vi "Drive Controller.vi"(8 "error in":errorcluster) -> ()   [LabVIEW 2017]
doc: "This VI executes continuously carrying out the current operation and responding to updates or new operation requests. It will often contain the timing or control code that is difficult to place directly in TeleOp. This VI generally opens all sensors and motors and isolates the rest of the robot code from knowing implementation details of how the operations are carried out."
uses:
  <vilib>/Rock Robotics/WPI/Framework/Completion Status.ctl
  Drive Setpoints.ctl
  Drive Operations.ctl
  Shared/RobotNeededPathData.ctl
  <vilib>/Rock Robotics/WPI/SafetyOutput/WPI_SafetyOutputConfigMenu.ctl
  <vilib>/Rock Robotics/SystemInterfaces/DIO/FPGA_DIOPWMChannel.ctl
  <vilib>/Rock Robotics/SystemInterfaces/DIO/FPGA_DIOChannel.ctl
  <vilib>/Rock Robotics/WPI/DriverStation/WPI_DriverStationRobotMode2.ctl
  <vilib>/Rock Robotics/WPI/ThirdParty/Sensors/navX/_TypeDefs/FRIC_navX_DeviceNumbersTypeDef.ctl
  <extravilib>/ChannelInstances/Lossy Stream-c(dbl,dbl,dbl,c(dbl,dbl))/Write With Abort.vi
  <extravilib>/ChannelInstances/Lossy Stream-c(dbl,dbl,dbl,c(dbl,dbl))/Read With Abort.vi
  <extravilib>/ChannelInstances/Lossy Stream-c(dbl,dbl,dbl,c(dbl,dbl))/Endpoint.vi
  <extravilib>/ChannelInstances/Lossy Stream-c(dbl,dbl,dbl,c(dbl,dbl))/EndpointRead.vi
  <vilib>/Rock Robotics/WPI/RobotDrive/WPI_RobotDriveOpen4MotorWithSPARK.vi
  <vilib>/Rock Robotics/WPI/Counter/WPI_CounterDigitalInputToDigitalSource.vi
  <vilib>/Rock Robotics/WPI/RobotDrive/WPI_RobotDriveOpen2MotorWithSPARK.vi
  <extravilib>/ChannelInstances/Lossy Stream-c(dbl,dbl,dbl,c(dbl,dbl))/Instantiate.vi
  <extravilib>/ChannelInstances/Lossy Stream-c(dbl,dbl,dbl,c(dbl,dbl))/)Channel.vi
  <resource>/ChannelSupport/_ChannelSupport/WaitIfNeeded.vi
  <vilib>/addons/control/pid/pid.llb/PID (DBL).vi
  Configuration/Constants.vi
  <vilib>/Rock Robotics/Network Tables/NT Read Number.vi
  Framework/Robot Global Data.vi
  Drive Published Globals.vi
  <vilib>/addons/control/pid/NI_PID_pid.lvlib
  <extravilib>/ChannelInstances/Lossy Stream-c(dbl,dbl,dbl,c(dbl,dbl)).lvlib
panel:
  out "Waveform Chart":cluster{dbl, dbl}(graph)={180.0, 177.43}
  in  "Points":cluster{"X":dbl, "Y":dbl}[](array[cluster])=[{"X"=0.0, "Y"=0.0}, {"X"=0.01, "Y"=0.0}, {"X"=0.011, "Y"=0.3}, {"X"=1.0, "Y"=1.0}]
  in  "PID gains":T1={"proportional gain (Kc)"=0.003, "integral time (Ti, min)"=0.0, "derivative time (Td, min)"=0.0} {"derivative time (Td, min)" format="%#_9g"}
  out "Numeric":dbl
  out "Yaw 2":dbl=2.309999999999988
  in  "Gains":T2={"FFV"=0.0059, "FFA"=0.0019, "Vel PID"={"P"=0.01, "I"=0.0, "D"=0.0}}
  in  "Interactive Values":T3={"Operation"=enum."Turn to Angle", "Left Speed"=-0.27, "Right Speed"=0.27, "Duration"=2.0, "Speed"=0.0, "Start Angle"=0.0, "Target Angle"=180.0, "Distance (inch)"=0.0, "Start Point (inch)"=0.0, "RobotNeededPathData"={"Path"=[], "MaxVel"=0.0, "MaxAccel"=-1.0, "Backwards?"=FALSE, "PointSpacing"=0.0, "LookaheadDist"=0.0, "Speed/Curve"=1.8, "SlowDistanceAtEnd"=12.0, "SlowSpeed"=15.0}} {"RobotNeededPathData"."SlowSpeed" format="%#_13g"; "RobotNeededPathData"."SlowDistanceAtEnd" format="%#_13g"; "RobotNeededPathData"."Speed/Curve" format="%#_13g"}
  in  "Buttons":cluster{"Execute Cmd":bool, "Abort Cmd":bool}
  out "Command Timing":cluster{"Start Time (ms)":u32, "Iterations":i32}={"Start Time (ms)"=1728587, "Iterations"=0}
  out "Status":T6
  out "Setpoints":T7(graph)
  out "Current\nCmd":string="Started at  15:35:35.928\nDefault: Reserve,  L 0.0, R 0.0, D 0.000000"
  # "Tip: The graph shows the motor setpoints. It may also be helpful to observe inputs and sensor values.\nYou may also want to display tuning or debugging controls."
  # ".0088"
  # ".0017"
  # ".02"
  # "Interactive Command: You may fill in the settings for a command\nand schedule it with the Execute button. You can observe and abort\nany command while fine tuning the code for the controller."
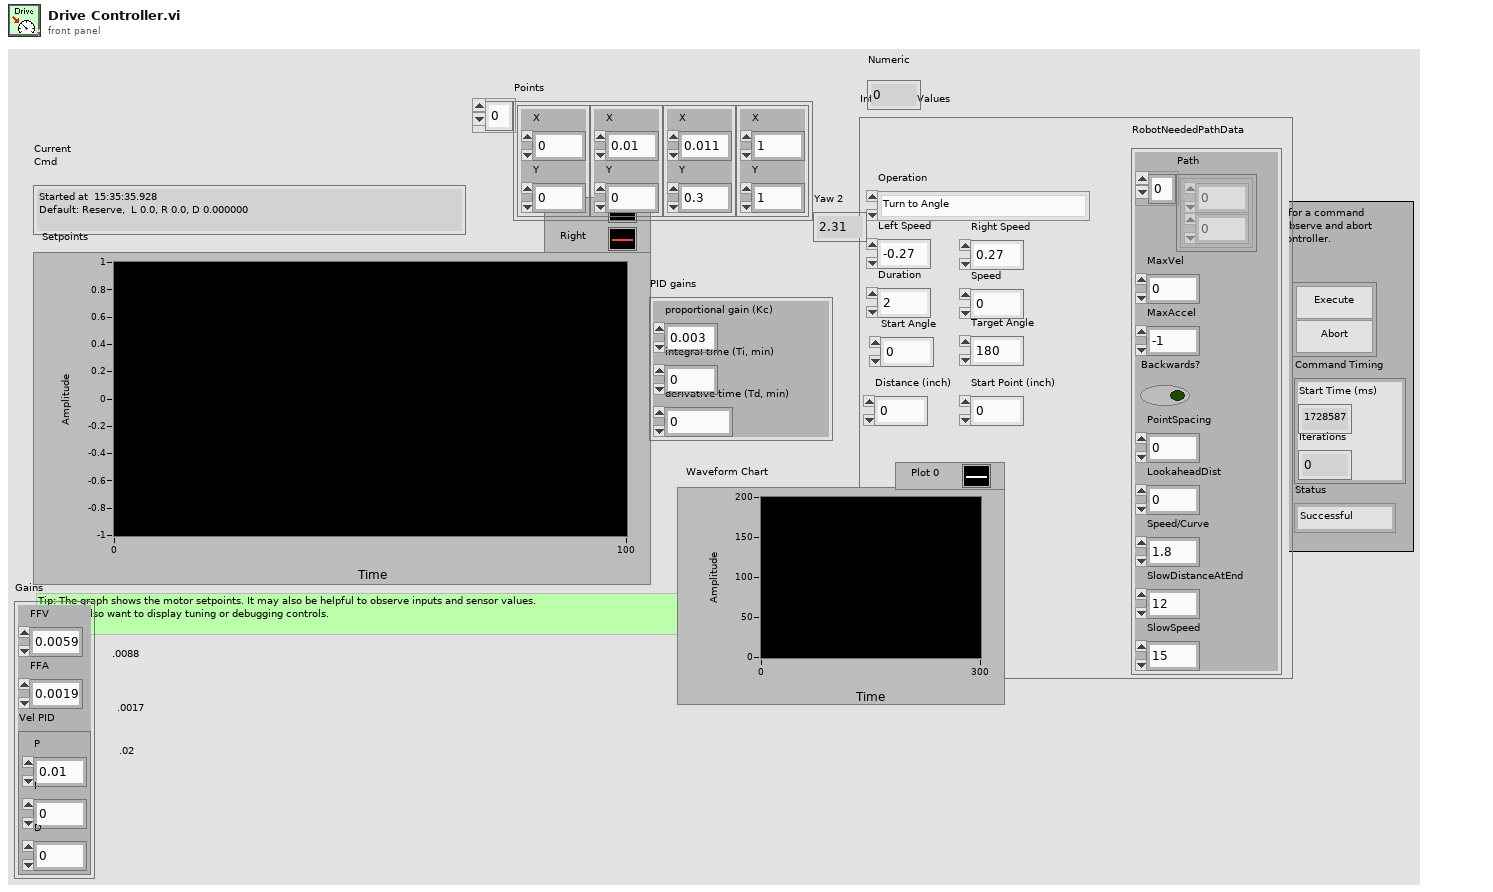
[diagram p1: front panel]
types:
  T1 = cluster{"proportional gain (Kc)":dbl, "integral time (Ti, min)":dbl, "derivative time (Td, min)":dbl}
  T2 = cluster{"FFV":dbl, "FFA":dbl, "Vel PID":cluster{"P":dbl, "I":dbl, "D":dbl}}
  T3 = typedef "Drive Setpoints.ctl" = cluster{"Operation":T4, "Left Speed":dbl, "Right Speed":dbl, "Duration":dbl, "Speed":dbl, "Start Angle":dbl, "Target Angle":dbl, "Distance (inch)":dbl, "Start Point (inch)":dbl, "RobotNeededPathData":T5}
  T4 = typedef "Drive Operations.ctl" = enum16{"Reserve", "Read Current", "Immediate", "Drive for Time", "Drive for Distance", "Turn to Angle", "Arc Turn", "Drive Path"}
  T5 = typedef "RobotNeededPathData.ctl" = cluster{"Path":cluster{dbl, dbl}[], "MaxVel":dbl, "MaxAccel":dbl, "Backwards?":bool, "PointSpacing":dbl, "LookaheadDist":dbl, "Speed/Curve":dbl, "SlowDistanceAtEnd":dbl, "SlowSpeed":dbl}
  T6 = typedef "Completion Status.ctl" = enum16{"Successful", "Aborted", "Incomplete"}
  T7 = cluster{"Left Setpoint":dbl, "Right Setpoint":dbl}
  T8 = typedef "FPGA_DIOChannel.ctl" = enum8{"DIO 0", "DIO 1", "DIO 2", "DIO 3", "DIO 4", "DIO 5", "DIO 6", "DIO 7", "DIO 8", "DIO 9", "DIO MXP 0", "DIO MXP 1", "DIO MXP 2", "DIO MXP 3", "DIO MXP 4", "DIO MXP 5", "DIO MXP 6", "DIO MXP 7", "DIO MXP 8", "DIO MXP 9", "DIO MXP 10", "DIO MXP 11", "DIO MXP 12", "DIO MXP 13", "DIO MXP 14", "DIO MXP 15", "SPI Port CS1", "SPI Port CS2", "SPI Port CS3", "SPI Port MISO", "SPI Port MOSI", "Invalid"}
  T9 = typedef "FPGA_DIOPWMChannel.ctl" = enum8{"PWM 0", "PWM 1", "PWM 2", "PWM 3", "PWM 4", "PWM 5", "PWM 6", "PWM 7", "PWM 8", "PWM 9", "PWM MXP 0", "PWM MXP 1", "PWM MXP 2", "PWM MXP 3", "PWM MXP 4", "PWM MXP 5", "PWM MXP 6", "PWM MXP 7", "PWM MXP 8", "PWM MXP 9", "Invalid"}
  T10 = typedef "WPI_SafetyOutputConfigMenu.ctl" = enum16{"Enable", "Disable"}
  T11 = typedef "WPI_DigitalInputDevRef.ctl" = cluster{"DevStatus":errorcluster, "DIO Channel":T8}
  T12 = typedef "FPGA_CounterEncoderSourceConvertionLVSourceType.ctl" = cluster{"DevStatus":errorcluster, "AnalogTriggerMode?":bool, "DigitalMode":cluster{"DIO Channel":T13}, "AnalogTriggerMode":cluster{"AnalogTriggerIndex":T14, "OutputType":T15}}
  T13 = typedef "FPGA_DIODigitalSourceChannel.ctl" = enum8{"DIO 0", "DIO 1", "DIO 2", "DIO 3", "DIO 4", "DIO 5", "DIO 6", "DIO 7", "DIO 8", "DIO 9", "DIO MXP 0", "DIO MXP 1", "DIO MXP 2", "DIO MXP 3", "DIO MXP 4", "DIO MXP 5", "DIO MXP 6", "DIO MXP 7", "DIO MXP 8", "DIO MXP 9", "DIO MXP 10", "DIO MXP 11", "DIO MXP 12", "DIO MXP 13", "DIO MXP 14", "DIO MXP 15", "Disabled"}
  T14 = typedef "FPGA_AnalogTriggerIndex.ctl" = enum8{"Trig 0", "Trig 1", "Trig 2", "Trig 3", "Trig 4", "Trig 5", "Trig 6", "Trig 7", "Invalid"}
  T15 = typedef "FPGA_AnalogTriggerOutType.ctl" = enum16{"InWindow", "TriggerState", "Rising", "Falling"}
  T16 = typedef "WPI_EncoderDevRef.ctl" = cluster{"DevStatus":errorcluster, "EncoderIndex":T17, "CounterIndex":T18, "DistancePerCount":dbl, "Decoding Type":T19}
  T17 = typedef "FPGA_EncoderIdx.ctl" = enum8{"Enc 0", "Enc 1", "Enc 2", "Enc 3", "Enc 4", "Enc 5", "Enc 6", "Enc 7", "Invalid"}
  T18 = typedef "FPGA_CounterCtrSystemIndex.ctl" = enum8{"Ctr 0", "Ctr 1", "Ctr 2", "Ctr 3", "Ctr 4", "Ctr 5", "Ctr 6", "Ctr 7", "Invalid"}
  T19 = typedef "WPI_EncoderType.ctl" = enum16{"1x", "2x", "4x"}
  T20 = typedef "WPI_RobotDriveDevRef.ctl" = cluster{"DevStatus":errorcluster, "Motors[]":T21[], "Square Inputs":bool, "Max Output":dbl}
  T21 = typedef "WPI_MotorControlDeviceRef.ctl" = cluster{"DeviceStatus":errorcluster, "Type":T22, "PWM":cluster{"PWM Channel":T9, "DeadBand":T23}, "CAN":cluster{"Device Number":u8, "SetOutput VI Ref":variant, "GetOutput VI Ref":variant, "Enable VI Ref":variant, "Disable VI Ref":variant, "Data":variant}, "Invert":bool, "DIO PWM":cluster{"PWM \"Enable\" Channel":T9, "DIOChannel":T8, "PWM Rate":dbl}}
  T22 = typedef "WPI_MotorControlType.ctl" = enum16{"PWM", "CAN", "DIO PWM"}
  T23 = typedef "WPI_PWMDeadband.ctl" = cluster{"Name":string, "maxPositivePwm":i32, "minPositivePwm":i32, "centerPwm":i32, "maxNegativePwm":i32, "minNegativePwm":i32, "angularRange":u16}
  T24 = typedef "Command Status Info.ctl" = cluster{"Name":string, "Status":T6, "notifier out":T25}
  T25 = typedef "Completion Notifier.ctl" = refnum<notifier>
  T26 = cluster{"SubSystem Data":T3, cluster{"Start Time (ms)":u32, "Iterations":i32}, cluster{"Command Info":T24, "Description":string, "Default Command":T3, "queue out":refnum<queue>, "Subsystem Name":string}}
  T27 = typedef "WPI_DriverStationRobotMode2.ctl" = enum16{"Autonomous Disabled", "Autonomous Enabled", "Teleop Disabled", "Teleop Enabled", "Disconnected", "Finish", "Test Disabled", "Test Enabled", "Emergency Stopped"}
  T28 = cluster{"Yaw":dbl, "Roll":dbl, "Pitch":dbl, "Heading":dbl, "Fused Heading":dbl}
  T29 = cluster{"dx/dt":dbl, "dx/dt":dbl, dbl, cluster{dbl, dbl}}
  T30 = typedef "Lossy Stream-c(dbl,dbl,dbl,c(dbl,dbl)).lvlib/)Channel.ctl" = refnum<queue>
  T31 = typedef "FRIC_navX_DeviceNumbersTypeDef.ctl" = enum16{"Dev0", "Dev1", "Dev2", "Dev3"}
  T32 = cluster{"LeftDistance":dbl, "RightDistance":dbl, "LeftVelocity":dbl, "RightVelocity":dbl, "Angle":dbl, "Location":cluster{dbl, dbl}}
  T33 = cluster{"dx/dt":dbl, "dx/dt":dbl, "Yaw":dbl, cluster{dbl, dbl}}
  T34 = cluster{"SubSystem Data":T3, cluster{"Start Time (ms)":u32, "Iterations":i32}, "Default Command Arguments":cluster{"Command Info":T24, "Description":string, "Default Command":T3, "queue out":refnum<queue>, "Subsystem Name":string}}
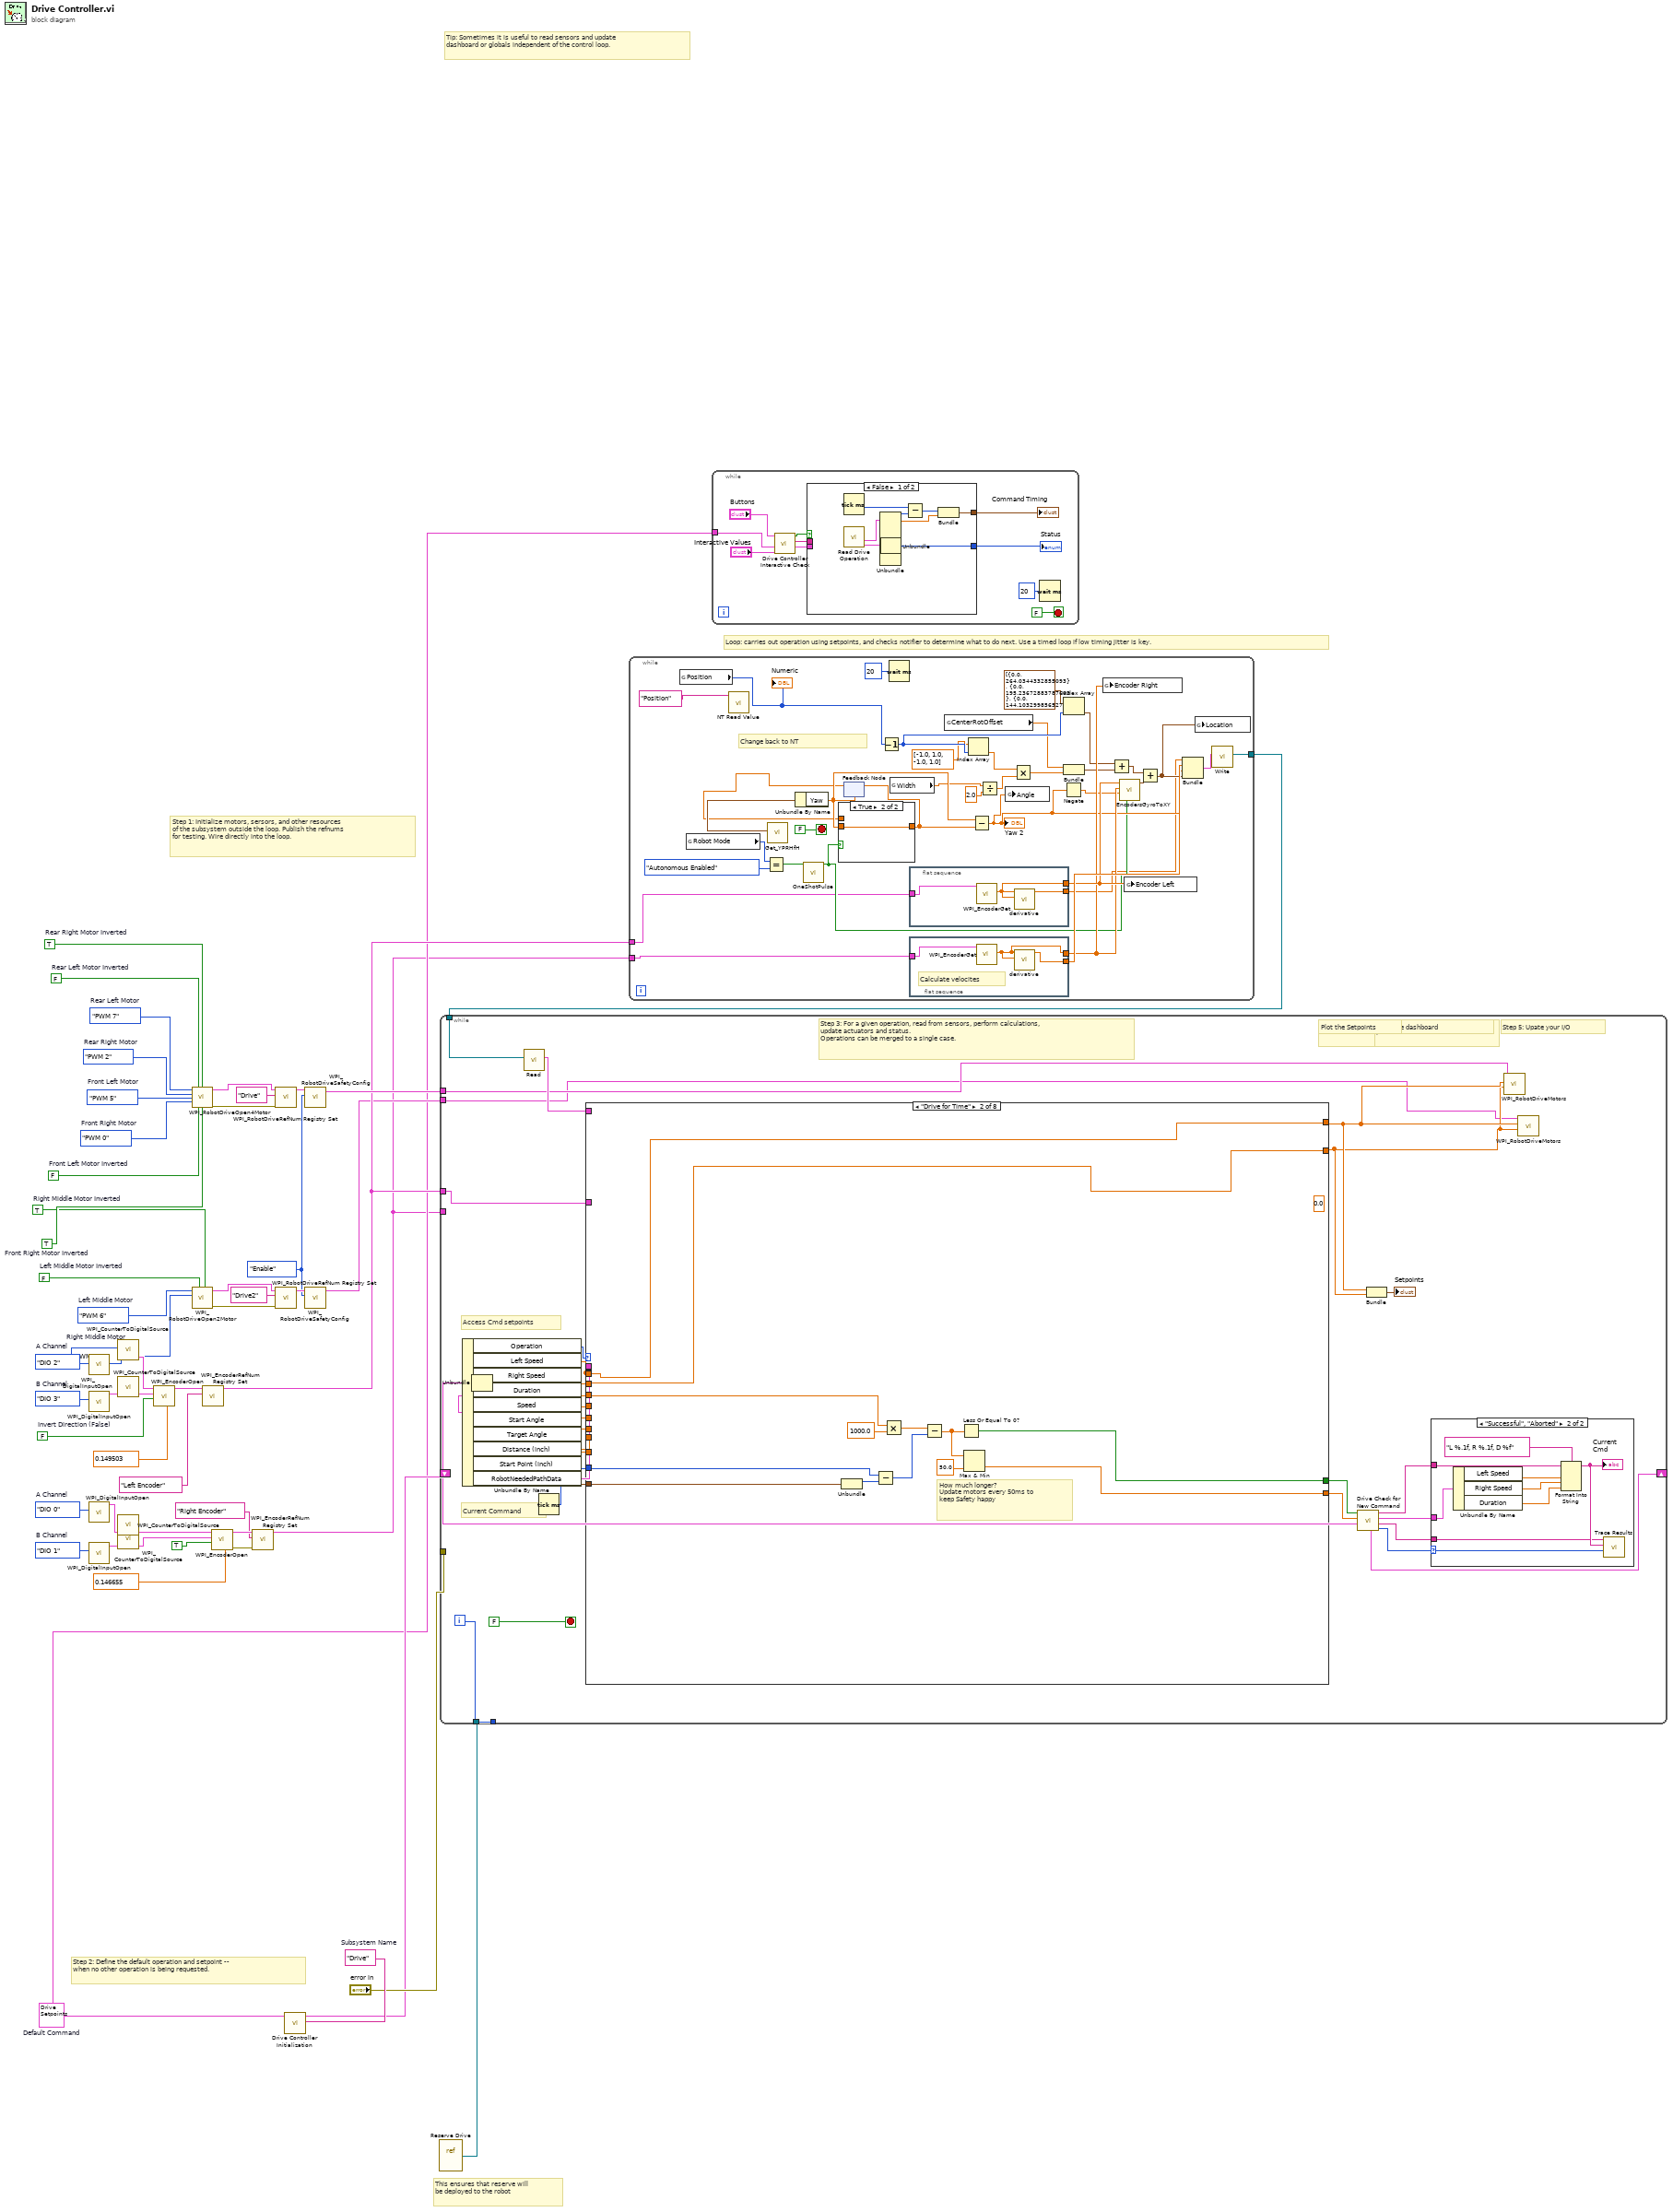
[diagram p0: block diagram]
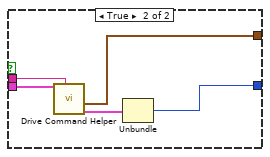
[diagram p3: hidden frame]
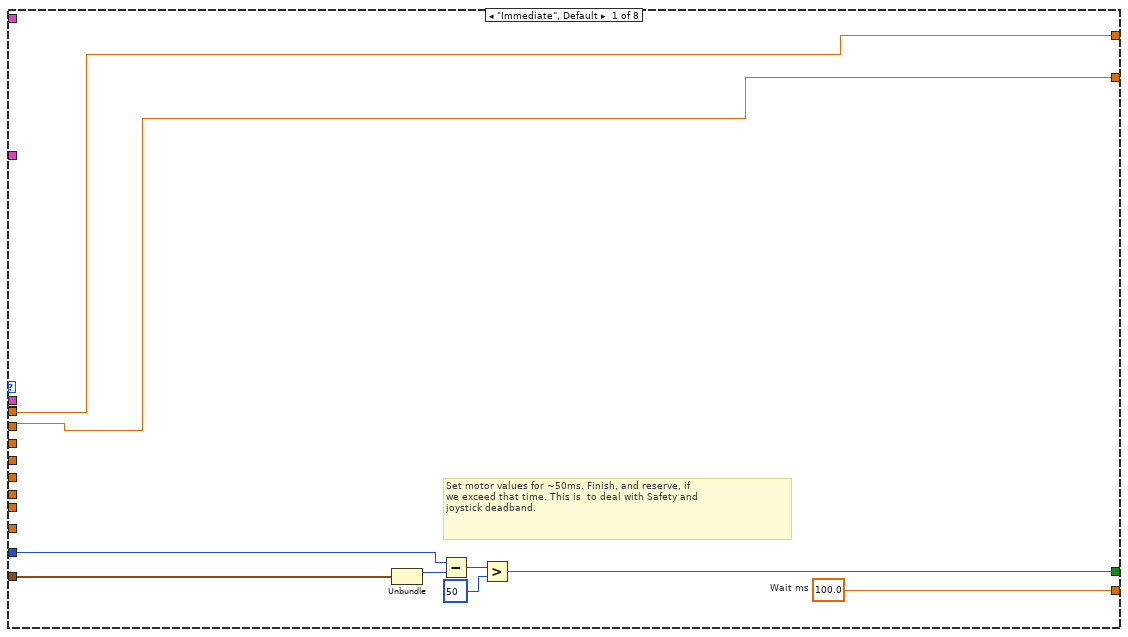
[diagram p4: hidden frame]
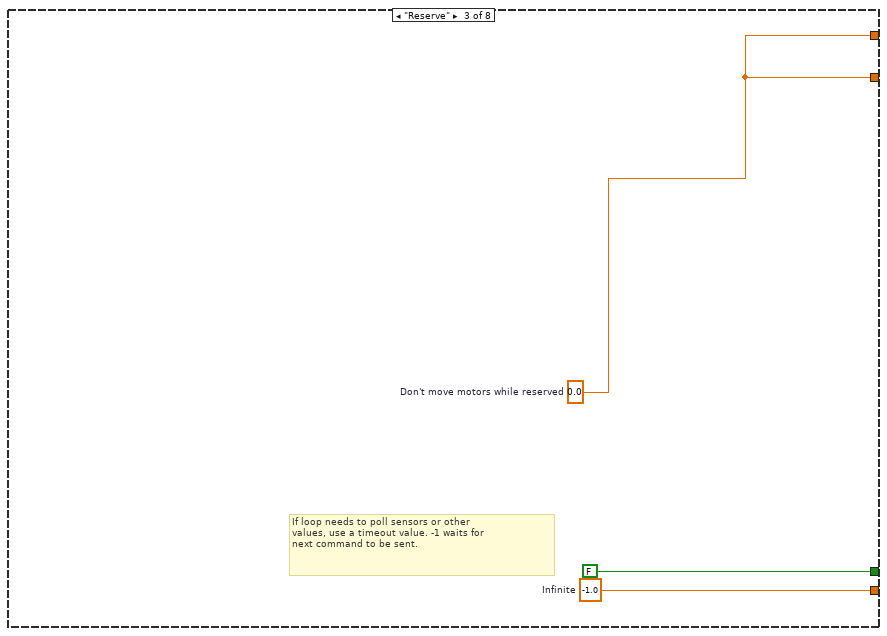
[diagram p5: hidden frame]
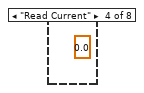
[diagram p6: hidden frame]
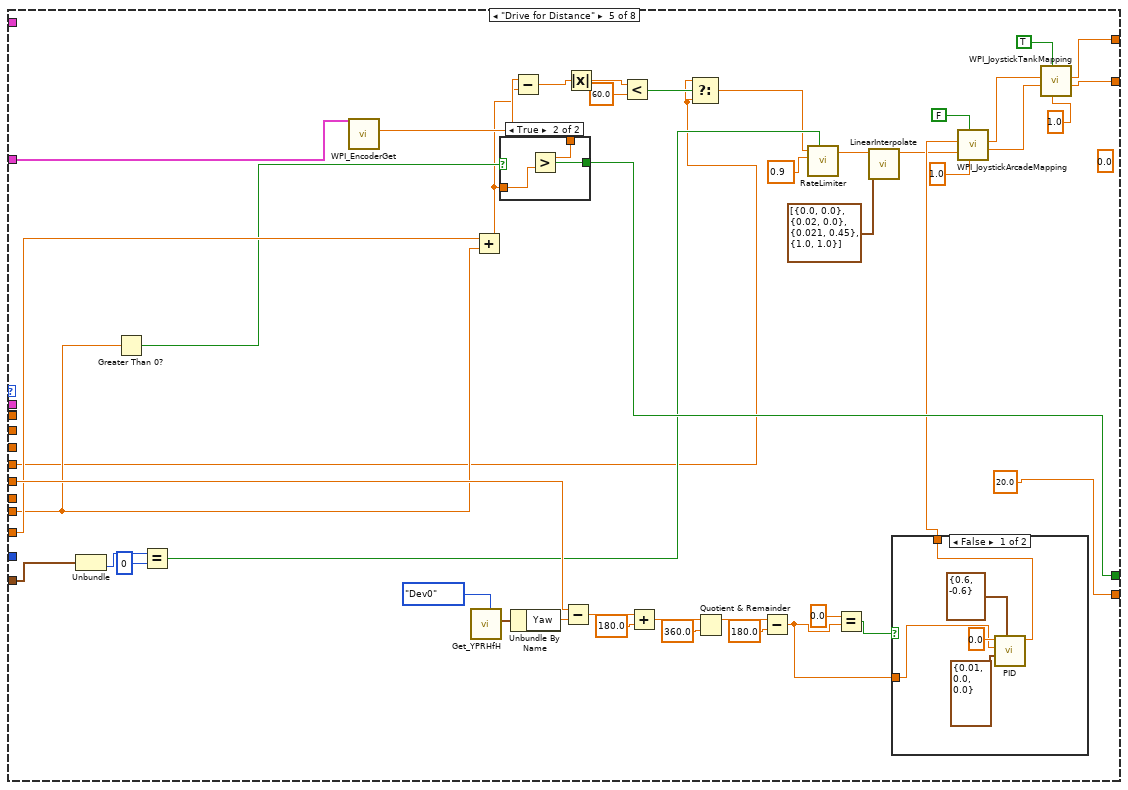
[diagram p7: hidden frame]
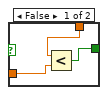
[diagram p8: hidden frame]
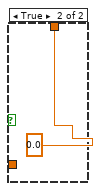
[diagram p9: hidden frame]
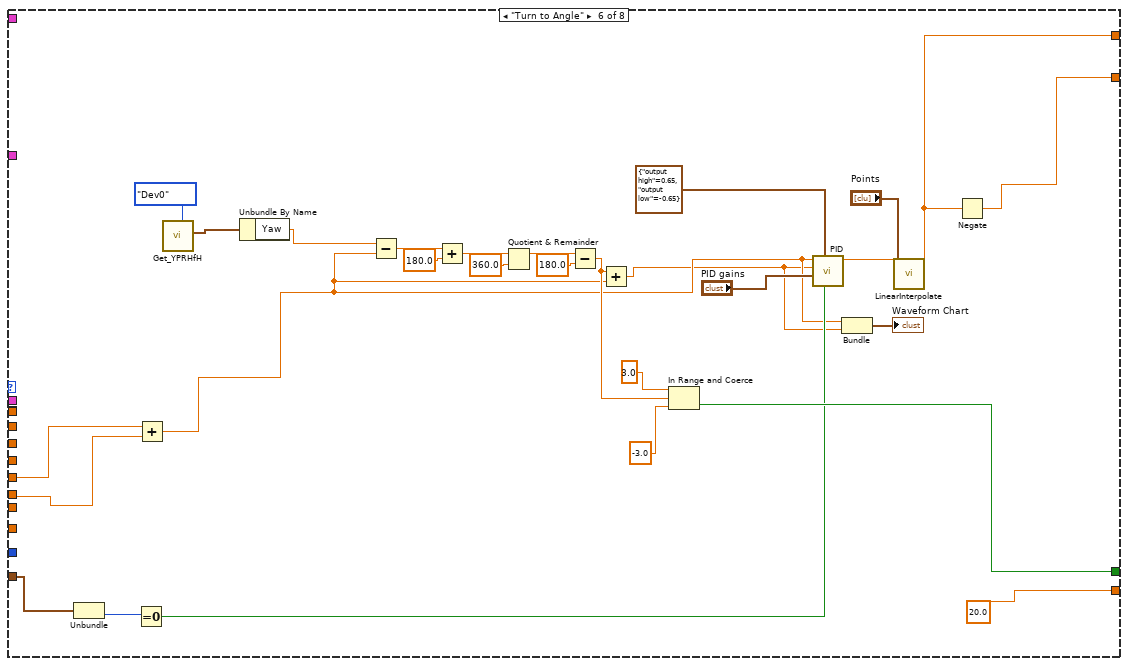
[diagram p10: hidden frame]
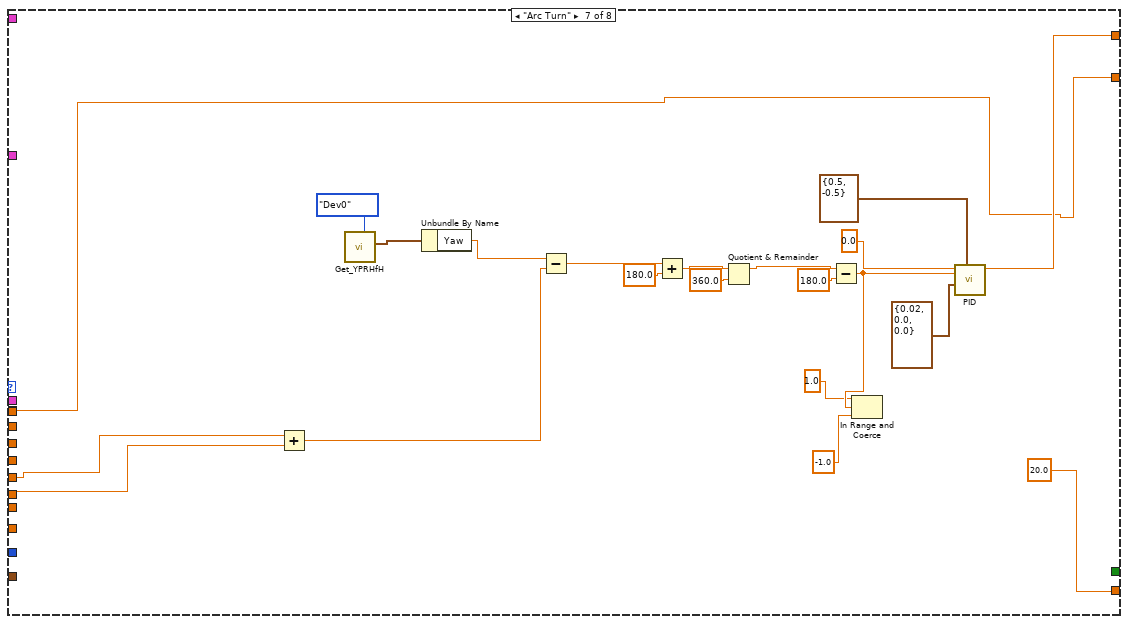
[diagram p11: hidden frame]
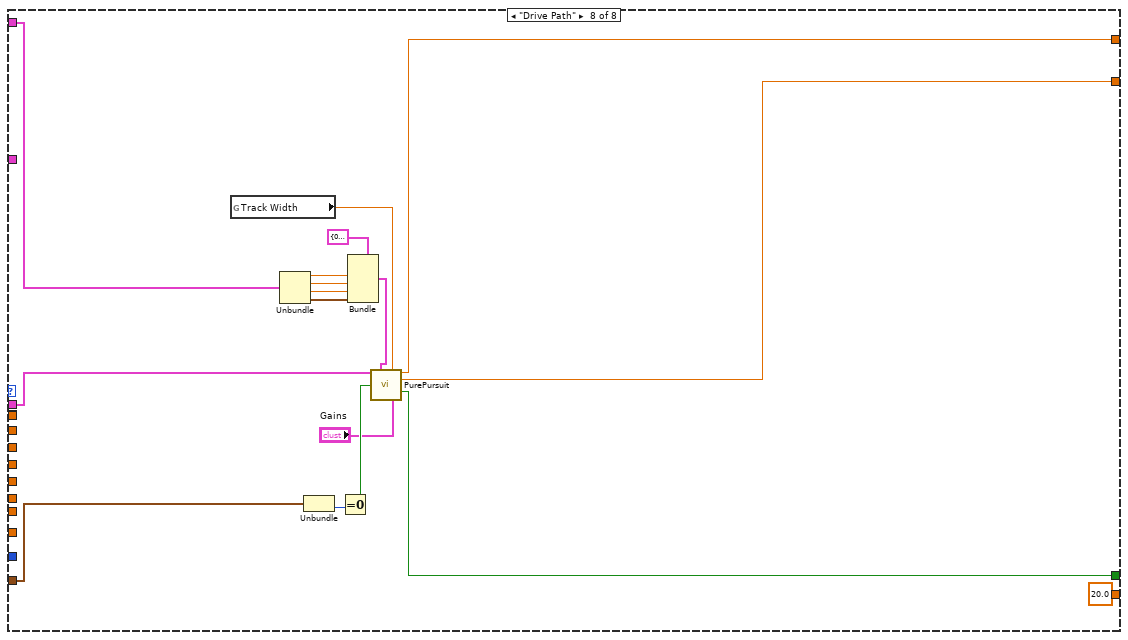
[diagram p12: hidden frame]
diagram:
  w4 = FPGA_DIOChannel."DIO 1"  # B Channel
  w7 = FPGA_DIOChannel."DIO 0"  # A Channel
  w14 = T3 {"Operation"=enum."Reserve", "Left Speed"=0.0, "Right Speed"=0.0, "Duration"=0.0, "Speed"=0.0, "Start Angle"=0.0, "Target Angle"=0.0, "Distance (inch)"=0.0, "Start Point (inch)"=0.0, "RobotNeededPathData"={"Path"=[], "MaxVel"=0.0, "MaxAccel"=0.0, "Backwards?"=FALSE, "PointSpacing"=0.0, "LookaheadDist"=0.0, "Speed/Curve"=1.8, "SlowDistanceAtEnd"=12.0, "SlowSpeed"=15.0}}  # Default Command
  w21 = TRUE  # Right Middle Motor Inverted
  w22 = FALSE  # Left Middle Motor Inverted
  w25 = FPGA_DIOPWMChannel."PWM 1"  # Right Middle Motor
  w26 = FPGA_DIOPWMChannel."PWM 6"  # Left Middle Motor
  w35 = FALSE  # Invert Direction (False)
  w28 = FPGA_DIOChannel."DIO 3"  # B Channel
  w29 = FPGA_DIOChannel."DIO 2"  # A Channel
  w37 = TRUE  # Front Right Motor Inverted
  w38 = FALSE  # Front Left Motor Inverted
  w39 = TRUE  # Rear Right Motor Inverted
  w40 = FALSE  # Rear Left Motor Inverted
  w41 = FPGA_DIOPWMChannel."PWM 0"  # Front Right Motor
  w42 = FPGA_DIOPWMChannel."PWM 5"  # Front Left Motor
  w43 = FPGA_DIOPWMChannel."PWM 2"  # Rear Right Motor
  w44 = FPGA_DIOPWMChannel."PWM 7"  # Rear Left Motor
  w16 = WPI_SafetyOutputConfigMenu."Enable" ("mode")
  w52 = "Drive"  # Subsystem Name
  # "Step 2: Define the default operation and setpoint --\nwhen no other operation is being requested."
  # "This ensures that reserve will\nbe deployed to the robot"
  # "Tip: Sometimes it is useful to read sensors and update\ndashboard or globals independent of the control loop."
  # "Step 1: Initialize motors, sersors, and other resources\nof the subsystem outside the loop. Publish the refnums\nfor testing. Wire directly into the loop."
  # "Loop: carries out operation using setpoints, and checks notifier to determine what to do next. Use a timed loop if low timing jitter is key."
  n1 = call <vilib>:"WPI_DigitalInputOpen.vi"("DIO Channel"=w29) -> ("DigitalInputDevRef"=w32:T11)  [unwired: 1 in, 9 out]
  n2 = call <vilib>:"WPI_DigitalInputOpen.vi"("DIO Channel"=w28) -> ("DigitalInputDevRef"=w31:T11)  [unwired: 1 in, 9 out]
  n3 = call <vilib>:"WPI_DigitalInputOpen.vi"("DIO Channel"=w7) -> ("DigitalInputDevRef"=w8:T11)  [unwired: 1 in, 9 out]
  n4 = call <vilib>:"WPI_DigitalInputOpen.vi"("DIO Channel"=w4) -> ("DigitalInputDevRef"=w5:T11)  [unwired: 1 in, 9 out]
  n5 = call-poly <vilib>:"WPI_CounterToDigitalSource.vi"("DigitalInputDevRef"=w32) -> ("Digital Source"=w33:T12)  [unwired: 6 out]
  n6 = call-poly <vilib>:"WPI_CounterToDigitalSource.vi"("DigitalInputDevRef"=w31) -> ("Digital Source"=w30:T12)  [unwired: 6 out]
  n7 = call-poly <vilib>:"WPI_CounterToDigitalSource.vi"("DigitalInputDevRef"=w8) -> ("Digital Source"=w9:T12)  [unwired: 6 out]
  n8 = call-poly <vilib>:"WPI_CounterToDigitalSource.vi"("DigitalInputDevRef"=w5) -> ("Digital Source"=w6:T12)  [unwired: 6 out]
  n9 = call <vilib>:"WPI_EncoderOpen.vi"("DistancePerCount"=0.149503, "Invert Direction (False)"=w35, "BSource"=w30, "ASource"=w33) -> ("EncoderDevRef"=w34:T16)  [unwired: 4 in, 3 out]
  n10 = call-poly <vilib>:"WPI_RobotDriveOpen4Motor.vi"("Rear Left Motor"=w44, "Rear Left Motor Inverted"=w40, "Rear Right Motor Inverted"=w39, "Rear Right Motor"=w43, "Front Left Motor"=w42, "Front Right Motor"=w41, "Front Left Motor Inverted"=w38, "Front Right Motor Inverted"=w37) -> ("RobotDriveDevRef"=w51:T20, "error out"=w49:errorcluster)  [unwired: 6 in]
  n11 = call-poly <vilib>:"WPI_RobotDriveOpen2Motor.vi"("Right Motor Inverted"=w21, "Left Motor Inverted"=w22, "Right Motor"=w25, "Left Motor"=w26) -> ("error out"=w20:errorcluster, "RobotDriveDevRef"=w24:T20)  [unwired: 6 in]
  n12 = call <vilib>:"WPI_EncoderRefNum Registry Set.vi"("refnum name"="Left Encoder", "EncoderDevRef"=w34) -> ("EncoderDevRef"=w27:T16)  [unwired: 8 in, 1 out]
  n13 = call <vilib>:"WPI_EncoderOpen.vi"("DistancePerCount"=0.146655, "Invert Direction (False)"=TRUE, "BSource"=w6, "ASource"=w9) -> ("error out"=w11:errorcluster, "EncoderDevRef"=w10:T16)  [unwired: 4 in, 2 out]
  n14 = call <vilib>:"WPI_EncoderRefNum Registry Set.vi"("error in (no error)"=w11, "refnum name"="Right Encoder", "EncoderDevRef"=w10) -> ("EncoderDevRef"=w12:T16)  [unwired: 7 in, 1 out]
  n15 = call <vilib>:"WPI_RobotDriveRefNum Registry Set.vi"("error in (no error)"=w49, "refnum name"="Drive", "RobotDriveDevRef"=w51) -> ("RobotDriveDevRef"=w19:T20)  [unwired: 1 in, 7 out]
  n16 = call <vilib>:"WPI_RobotDriveRefNum Registry Set.vi"("error in (no error)"=w20, "refnum name"="Drive2", "RobotDriveDevRef"=w24) -> ("RobotDriveDevRef"=w18:T20)  [unwired: 7 in, 1 out]
  n17 = call "Drive Controller Initialization.vi"("Subsystem Name"=w52, "Default Command"=w14) -> ("Current Command"=w46:T26)  [unwired: 9 in]
  n18 = call <vilib>:"WPI_RobotDriveSafetyConfig.vi"("mode"=w16, "RobotDriveDevRef"=w19) -> ("RobotDriveDevRef"=w48:T20)  [unwired: 8 in, 1 out]
  n19 = call <vilib>:"WPI_RobotDriveSafetyConfig.vi"("mode"=w16, "RobotDriveDevRef"=w18) -> ("RobotDriveDevRef"=w17:T20)  [unwired: 8 in, 1 out]
  n20 = vi-ref "Reserve Drive.vi"() -> (w45:refnum<vi>)
  n21 = while {
    tunnel: [w57] -> w13
    tunnel: w12 -> [w56]
    tunnel: w27 -> [w55]
    stop <- FALSE stop-if-true
    # "Change back to NT"
    n22 = global read "Robot Global Data.vi" "Position"() -> (w53:u32)
    "Numeric" <- w53
    n23 = global read "Robot Global Data.vi" "Robot Mode"() -> (w72:T27)
    n24 = call-poly <vilib>:"NT Read Value.vi"("Name"="Position") -> ()  [unwired: 9 in, 2 out]
    n25 = Equal?(x=w72, y=WPI_DriverStationRobotMode2."Autonomous Enabled") -> (x = y?=w73:bool)
    n26 = call <vilib>:"Get_YPRHfH.vi"() -> ("YRPHfH"=w88:T28)  [unwired: 11 in]
    n27 = Unbundle By Name(w88) -> ("Yaw"=w76:dbl)
    n28 = call "OneShotPulse.vi"("Input"=w73) -> ("Output"=w74:bool)  [unwired: 10 in]
    n29 = feedback #1(w76) -> (w75:dbl)
    n30 = case shown="True" w74 {
      tunnel: w76 -> [_ w93]
      tunnel: [w92 w93] -> w77
      tunnel: w75 -> [w92 _]
      frame False {
      }
      frame True {
      }
    }
    n31 = feedback-in #1(w77) -> ()
    n32 = Decrement(x=w53) -> (x-1=w66:u32)
    n33 = Wait (ms)(milliseconds to wait=u32 20) -> ()  [unwired: 1 out]
    n34 = global read "Constants.vi" "Width"() -> (w61:dbl)
    n35 = flat-sequence {
      tunnel: [w91] -> w58
      tunnel: [w90] -> w81
      tunnel: w55 -> [w89]
      frame #0 {
        n36 = call <vilib>:"WPI_EncoderGet.vi"("EncoderDevRef"=w89) -> ("Distance"=w90:dbl)  [unwired: 5 in, 5 out]
        n37 = call "derivative.vi"("Starting value"=w90, "x"=w90) -> ("dx/dt"=w91:dbl)  [unwired: 9 in]
      }
    }
    n38 = flat-sequence {
      tunnel: [w95] -> w85
      tunnel: [w94] -> w80
      tunnel: w56 -> [w96]
      frame #0 {
        # "Calculate velocites"
        n39 = call <vilib>:"WPI_EncoderGet.vi"("EncoderDevRef"=w96) -> ("Distance"=w94:dbl)  [unwired: 5 in, 5 out]
        n40 = call "derivative.vi"("Starting value"=w94, "x"=w94) -> ("dx/dt"=w95:dbl)  [unwired: 9 in]
      }
    }
    n41 = global read "Constants.vi" "CenterRotOffset"() -> (w59:dbl)
    n42 = Index Array(array=dbl[] [-1.0, 1.0, -1.0, 1.0], index=w66) -> (element=w67:dbl)
    n43 = Subtract(x=w76, y=w77) -> (x-y=w78:dbl)
    "Yaw 2" <- w78
    n44 = Divide(x=w61, y=2.0) -> (x/y=w62:dbl)
    n45 = global write "Drive Published Globals.vi" "Angle"(w78) -> ()
    n46 = Multiply(x=w67, y=w62) -> (x*y=w68:dbl)
    n47 = Negate(x=w78) -> (-x=w79:dbl)
    n48 = Index Array(array=cluster{dbl, dbl}[] [{0.0, 264.0344332855093}, {0.0, 195.23672883787663}, {0.0, 144.10329985652797}, {0.0, -0.0}] ("x*y"), index=w66) -> (element=w65:cluster{dbl, dbl})
    n49 = Bundle("CenterRotOffset"=w59, w68) -> (w69:cluster{"CenterRotOffset":dbl, dbl})  [unwired: 1 in]
    n50 = global write "Drive Published Globals.vi" "Encoder Right"(w80) -> ()
    n51 = Add(x=w65, y=w69) -> (x+y=w70:cluster{dbl, dbl})
    n52 = call "EncodersGyroToXY.vi"("Reset"=w74, "Angle (degrees)"=w79, "Right Distance"=w80, "Left Distance"=w81) -> ("Location"=w82:cluster{dbl, dbl})  [unwired: 7 in]
    n53 = global write "Drive Published Globals.vi" "Encoder Left"(w81) -> ()
    n54 = Add(x=w70, y=w82) -> (x+y=w83:cluster{dbl, dbl})
    n55 = Bundle("dx/dt"=w58, "dx/dt"=w85, w78, w83) -> (w84:T29)  [unwired: 1 in]
    n56 = global write "Drive Published Globals.vi" "Location"(w83) -> ()
    n57 = call <extravilib>:"Write.vi"("element"=w84) -> ("channel"=w57:T30)  [unwired: 8 in, 2 out]
  }
  n58 = while {
    shift-right: [w123] -> _
    shift-left: w46 -> [w116]
    tunnel: [w126] -> _
    tunnel: w48 -> [w99]
    tunnel: "error in" -> [_]
    tunnel: w45 -> [_]
    tunnel: w27 -> [w97]
    tunnel: w17 -> [w98]
    tunnel: w13 -> [w101]
    tunnel: w12 -> [_]
    i -> [w126]
    stop <- FALSE stop-if-true
    # "Plot the Setpoints"
    # "Step 5: Upate your I/O"
    # "Step 4: Format a string to describe this\ncmd and how the previous cmd finished"
    # "Current Command"
    # "Update motors and update dashboard"
    # "Access Cmd setpoints"
    # "Finished? &\nWait Time"
    # "Step 3: For a given operation, read from sensors, perform calculations,\nupdate actuators and status.\nOperations can be merged to a single case."
    n59 = Unbundle(w116) -> ("SubSystem Data"=w102:T3, w117:cluster{"Start Time (ms)":u32, "Iterations":i32})  [unwired: 1 out]
    n60 = Unbundle By Name(w102) -> ("Operation"=w112:T4, "Left Speed"=w111:dbl, "Right Speed"=w110:dbl, "Duration"=w109:dbl, "Speed"=w108:dbl, "Start Angle"=w107:dbl, "Target Angle"=w106:dbl, "Distance (inch)"=w105:dbl, "Start Point (inch)"=w104:dbl, "RobotNeededPathData"=w103:T5)
    n61 = call <extravilib>:"Read.vi"("channel"=w101) -> ("element"=w100:T33)  [unwired: 5 in, 5 out]
    n62 = Tick Count (ms)() -> (millisecond timer value=w125:u32)
    n63 = case shown="\"Drive for Time\"" w112 {
      tunnel: [w136 w140 w152 _ 20.0 ("Infinite") 20.0 ("Infinite") 20.0 ("Infinite") 20.0 ("Infinite")] -> w122
      tunnel: [w131 w144 FALSE ("ignore previous (F)") _ w184 w227 _ w271] -> w121
      tunnel: w117 -> [w130 w146 _ _ w164 w216 _ w261]
      tunnel: w125 -> [w132 w143 _ _ _ _ _ _]
      tunnel: [w129 w138 w150 _ w169 w213 w238 w273] -> w114
      tunnel: [w128 w137 w150 _ w170 w212 w237 w272] -> w113
      tunnel: w108 -> [_ _ _ _ w153 _ _ _]
      tunnel: w105 -> [_ _ _ _ w176 _ _ _]
      tunnel: w109 -> [_ w139 _ _ _ _ _ _]
      tunnel: w111 -> [w129 _ _ _ _ _ w237 _]
      tunnel: w110 -> [w128 w137 _ _ _ _ _ _]
      tunnel: w97 -> [_ _ _ _ w182 _ _ _]
      tunnel: w107 -> [_ _ _ _ w178 w230 w241 _]
      tunnel: w106 -> [_ _ _ _ _ w229 w240 _]
      tunnel: w104 -> [_ _ _ _ w177 _ _ _]
      tunnel: w111 -> [_ w138 _ _ _ _ _ _]
      tunnel: w103 -> [_ _ _ _ _ _ _ w274]
      tunnel: w100 -> [_ _ _ _ _ _ _ w265]
      frame "Immediate", Default {
        w136 = 100.0  # Wait ms
        # "Set motor values for ~50ms. Finish, and reserve, if\nwe exceed that time. This is  to deal with Safety and\njoystick deadband."
        n64 = Unbundle(w130) -> ("Start Time (ms)"=w133:u32)  [unwired: 1 out]
        n65 = Subtract(x=w132, y=w133) -> (x-y=w134:u32)
        n66 = Greater?(x=w134, y=u8 50 ("Left Motor")) -> (0:w131:bool)
      }
      frame "Drive for Time" {
        (unwired) 0.0 ("output")
        # "How much longer?\nUpdate motors every 50ms to\nkeep Safety happy"
        n67 = Unbundle(w146) -> ("Start Time (ms)"=w145:u32)  [unwired: 1 out]
        n68 = Subtract(x=w143, y=w145) -> (x-y=w149:u32)
        n69 = Multiply(x=w139, y=1000.0) -> (x*y=w148:dbl)
        n70 = Subtract(x=w148, y=w149) -> (x-y=w142:dbl)
        n71 = Less Or Equal To 0?(x=w142) -> (x <= 0?=w144:bool)
        n72 = Max & Min(x=w142, y=50.0) -> (min(x,y)=w140:dbl)  [unwired: 1 out]
      }
      frame "Reserve" {
        w150 = 0.0  # Don't move motors while reserved
        w152 = -1.0  # Infinite
        # "If loop needs to poll sensors or other\nvalues, use a timeout value. -1 waits for\nnext command to be sent."
      }
      frame "Read Current" {
        (unwired) 0.0 ("output")
      }
      frame "Drive for Distance" {
        (unwired) 0.0 ("output")
        n73 = Unbundle(w164) -> ("Iterations"=w163:i32)  [unwired: 1 out]
        n74 = Greater Than 0?(x=w176) -> (x > 0?=w175:bool)
        n75 = Equal?(x=w163, y=0) -> (x = y?=w161:bool)
        n76 = call <vilib>:"WPI_EncoderGet.vi"("EncoderDevRef"=w182) -> ("Distance"=w160:dbl)  [unwired: 5 in, 5 out]
        n77 = call <vilib>:"Get_YPRHfH.vi"("Device Number"=FRIC_navX_DeviceNumbersTypeDef."Dev0") -> ("YRPHfH"=w196:T28)  [unwired: 10 in]
        n78 = Add(x=w177, y=w176) -> (x+y=w159:dbl)
        n79 = case shown="True" w175 {
          tunnel: w160 -> [w198 w202]
          tunnel: w159 -> [w199 w201]
          tunnel: [w197 w200] -> w184
          frame False {
            n80 = Less?(x=w198, y=w199) -> (x < y?=w197:bool)
          }
          frame True {
            n81 = Greater?(x=w202, y=w201) -> (0:w200:bool)
          }
        }
        n82 = Unbundle By Name(w196) -> ("Yaw"=w187:dbl)
        n83 = Subtract(x=w160, y=w159) -> (x-y=w158:dbl)
        n84 = Subtract(x=w178, y=w187) -> (x-y=w186:dbl)
        n85 = Absolute Value(x=w158) -> (abs(x)=w157:dbl)
        n86 = Less?(x=w157, y=60.0) -> (x < y?=w155:bool)
        n87 = Add(x=w186, y=180.0) -> (x+y=w191:dbl)
        n88 = Select(t=w153, s=w155, f=w153) -> (s? t:f=w154:dbl)
        n89 = Quotient & Remainder(x=w191, y=360.0) -> (x-y*floor(x/y)=w189:dbl)  [unwired: 1 out]
        n90 = Subtract(x=w189, y=180.0) -> (x-y=w185:dbl)
        n91 = call "RateLimiter.vi"("Reset"=w161, "Max dx/dt"=0.9, "Input"=w154) -> ("Output"=w172:dbl)  [unwired: 8 in]
        n92 = Equal?(x=0.0, y=w185) -> (x = y?=w194:bool)
        n93 = call "LinearInterpolate.vi"("Points"=cluster{"X":dbl, "Y":dbl}[] [{"X"=0.0, "Y"=0.0}, {"X"=0.02, "Y"=0.0}, {"X"=0.021, "Y"=0.45}, {"X"=1.0, "Y"=1.0}], "Value"=w172) -> ("Output"=w173:dbl)  [unwired: 9 in]
        n94 = case shown="False" w194 {
          tunnel: [w203 0.0] -> w179
          tunnel: w185 -> [w204 _]
          frame False {
            n95 = call-poly <vilib>:"PID.vi"("output range"=cluster{"output high":dbl, "output low":dbl} {"output high"=0.6, "output low"=-0.6}, "PID gains"=T1 {"proportional gain (Kc)"=0.01, "integral time (Ti, min)"=0.0, "derivative time (Td, min)"=0.0}, "process variable"=w204, "setpoint"=0.0) -> ("output"=w203:dbl)  [unwired: 6 in, 1 out]
          }
          frame True {
          }
        }
        n96 = call <vilib>:"WPI_JoystickArcadeMapping.vi"("Max Output"=1.0, "Square Inputs"=FALSE, "Y axis value"=w173, "X axis value"=w179) -> ("Right Motor Value"=w168:dbl, "Left Motor Value"=w167:dbl)  [unwired: 6 in]
        n97 = call <vilib>:"WPI_JoystickTankMapping.vi"("Max Output"=1.0, "Square Inputs"=TRUE, "Right axis value"=w168, "Left axis value"=w167) -> ("Right Motor Value"=w170:dbl, "Left Motor Value"=w169:dbl)  [unwired: 6 in]
      }
      frame "Turn to Angle" {
        n98 = Unbundle(w216) -> ("Iterations"=w215:i32)  [unwired: 1 out]
        n99 = Equal To 0?(x=w215) -> (x = 0?=w214:bool)
        n100 = Add(x=w230, y=w229) -> (x+y=w211:dbl)
        n101 = call <vilib>:"Get_YPRHfH.vi"("Device Number"=FRIC_navX_DeviceNumbersTypeDef."Dev0") -> ("YRPHfH"=w232:T28)  [unwired: 10 in]
        n102 = Unbundle By Name(w232) -> ("Yaw"=w220:dbl)
        n103 = Subtract(x=w220, y=w211) -> (x-y=w221:dbl)
        n104 = Add(x=w221, y=180.0) -> (x+y=w224:dbl)
        n105 = Quotient & Remainder(x=w224, y=360.0) -> (x-y*floor(x/y)=w222:dbl)  [unwired: 1 out]
        n106 = Subtract(x=w222, y=180.0) -> (x-y=w219:dbl)
        n107 = Add(x=w219, y=w211) -> (x+y=w210:dbl)
        n108 = In Range and Coerce(upper limit=3.0, x=w219, lower limit=-3.0) -> (In Range?=w227:bool)  [unwired: 1 out]
        n109 = call-poly <vilib>:"PID.vi"("reinitialize? (F)"=w214, "output range"=cluster{"output high":dbl, "output low":dbl} {"output high"=0.65, "output low"=-0.65}, "PID gains"="PID gains", "process variable"=w210, "setpoint"=w211) -> ("output"=w218:dbl)  [unwired: 5 in, 1 out]
        n110 = Bundle(w211, w210) -> (→"Waveform Chart":cluster{dbl, dbl})  [unwired: 1 in]
        n111 = call "LinearInterpolate.vi"("Points"="Points", "Value"=w218) -> ("Output"=w213:dbl)  [unwired: 9 in]
        n112 = Negate(x=w213) -> (-x=w212:dbl)
      }
      frame "Arc Turn" {
        n113 = Add(x=w241, y=w240) -> (x+y=w248:dbl)
        n114 = call <vilib>:"Get_YPRHfH.vi"("Device Number"=FRIC_navX_DeviceNumbersTypeDef."Dev0") -> ("YRPHfH"=w244:T28)  [unwired: 10 in]
        n115 = Unbundle By Name(w244) -> ("Yaw"=w242:dbl)
        n116 = Subtract(x=w242, y=w248) -> (x-y=w250:dbl)
        n117 = Add(x=w250, y=180.0) -> (x+y=w253:dbl)
        n118 = Quotient & Remainder(x=w253, y=360.0) -> (x-y*floor(x/y)=w251:dbl)  [unwired: 1 out]
        n119 = Subtract(x=w251, y=180.0) -> (x-y=w247:dbl)
        n120 = In Range and Coerce(upper limit=1.0, x=w247, lower limit=-1.0) -> ()  [unwired: 2 out]
        n121 = call-poly <vilib>:"PID.vi"("output range"=cluster{"output high":dbl, "output low":dbl} {"output high"=0.5, "output low"=-0.5}, "PID gains"=T1 {"proportional gain (Kc)"=0.02, "integral time (Ti, min)"=0.0, "derivative time (Td, min)"=0.0}, "process variable"=w247, "setpoint"=0.0) -> ("output"=w238:dbl)  [unwired: 6 in, 1 out]
      }
      frame "Drive Path" {
        n122 = global read "Constants.vi" "Track Width"() -> (w260:dbl)
        n123 = Unbundle(w265) -> ("dx/dt"=w269:dbl, "dx/dt"=w268:dbl, "Yaw"=w267:dbl, w266:cluster{dbl, dbl})
        n124 = Unbundle(w261) -> ("Iterations"=w262:i32)  [unwired: 1 out]
        n125 = Equal To 0?(x=w262) -> (x = 0?=w263:bool)
        n126 = Bundle(cluster=T32 {"LeftDistance"=0.0, "RightDistance"=0.0, "LeftVelocity"=0.0, "RightVelocity"=0.0, "Angle"=0.0, "Location"={0.0, 0.0}} ("SensorData"), "LeftVelocity"=w269, "RightVelocity"=w268, "Angle"=w267, "Location"=w266) -> (w270:T32)  [unwired: 2 in]
        n127 = call "PurePursuit.vi"("RobotNeededPathData"=w274, "SensorData"=w270, "Trackwidth"=w260, "Reset"=w263, "Gains"="Gains") -> ("LeftValue"=w273:dbl, "RightValue"=w272:dbl, "Done"=w271:bool)  [unwired: 6 in, 2 out]
      }
    }
    n128 = call "Drive Check for New Command.vi"("input cluster"=w116, "Wait time (ms)"=w122, "Finished?"=w121) -> ("Completion"=w124:T6, "Subsystem Name"=w118:string, "Current Command"=w119:T3, "Initial Trace String"=w120:string, "Next Command"=w123:T34)  [unwired: 4 in]
    n129 = Bundle("LeftValue"=w114, "RightValue"=w113) -> (→"Setpoints":cluster{"LeftValue":dbl, "RightValue":dbl})  [unwired: 1 in]
    n130 = case shown="\"Successful\", \"Aborted\"" w124 {
      selector: w124 -> [_ w283]
      tunnel: w120 -> [_ w278]
      tunnel: w119 -> [_ w279]
      tunnel: w118 -> [_ w275]
      frame "Incomplete", Default {
        # "Continuing current command"
      }
      frame "Successful", "Aborted" {
        # "Report and setup for next command"
        n131 = Unbundle By Name(w279) -> ("Left Speed"=w281:dbl, "Right Speed"=w282:dbl, "Duration"=w276:dbl)
        n132 = Format Into String(format string="L %.1f, R %.1f, D %f", initial string=w278, w281, w282, w276) -> (resulting string=w277:string)  [unwired: 1 in, 1 out]
        "Current\nCmd" <- w277
        n133 = call <vilib>:"Trace Results.vi"("Status of previous command"=w283, "Description"=w277, "Subsystem"=w275) -> ()  [unwired: 9 in]
      }
    }
    n134 = call <vilib>:"WPI_RobotDriveMotors.vi"("RightSpeed"=w113, "LeftSpeed"=w114, "RobotDriveDevRef"=w99) -> ()  [unwired: 1 in, 8 out]
    n135 = call <vilib>:"WPI_RobotDriveMotors.vi"("RightSpeed"=w113, "LeftSpeed"=w114, "RobotDriveDevRef"=w98) -> ()  [unwired: 1 in, 8 out]
  }
  n136 = while {
    tunnel: w14 -> [w285]
    stop <- FALSE stop-if-true
    n137 = call "Drive Controller Interactive Check.vi"("Interactive Command In"="Interactive Values", "Default Command"=w285, "Buttons"="Buttons") -> ("Interactive Command Out"=w287:T3, "Trace String"=w288:string, "Schedule"=w289:bool)  [unwired: 6 in]
    n138 = case shown="False" w289 {
      tunnel: [w298 w306] -> w290
      tunnel: [w297 w302] -> w291
      tunnel: w288 -> [_ w304]
      tunnel: w287 -> [_ w303]
      frame False {
        n139 = Tick Count (ms)() -> (millisecond timer value=w301:u32)
        n140 = call "Read Drive Operation.vi"() -> ("Command Info"=w295:T24, "SubSystem Data"=w294:T3)  [unwired: 9 in, 1 out]
        n141 = Unbundle(w294) -> ("Operation"=w299:T4, "Left Speed"=w296:dbl)  [unwired: 8 out]
        n142 = Unbundle(w295) -> ("Status"=w298:T6)  [unwired: 2 out]
        n143 = Subtract(x=w301, y=w299) -> (x-y=w300:u32)
        n144 = Bundle(w300, "Left Speed"=w296) -> (w297:cluster{u32, "Left Speed":dbl})  [unwired: 1 in]
      }
      frame True {
        n145 = call "Drive Command Helper.vi"("Description"=w304, "SubSystem Data"=w303) -> ("Command Info Out"=w305:T24, "Command Timing"=w302:cluster{"Start Time (ms)":u32, "Iterations":i32})  [unwired: 7 in, 1 out]
        n146 = Unbundle(w305) -> ("Status"=w306:T6)  [unwired: 2 out]
      }
    }
    "Status" <- w290
    "Command Timing" <- w291
    n147 = Wait (ms)(milliseconds to wait=u32 20) -> ()  [unwired: 1 out]
  }
